vi "Generator.vi"() -> ()   [LabVIEW 2018]
uses:
  <instrlib>/Siglent SDG X Series/Siglent SDG X Series.lvlib
panel:
  in  "Filename":string="1"
  in  "File Directory":path
  out "Output Directory":path
  in  "format string":string="Channel: %g \nWavetype: %g \nAMP: %gV\nFreq: %gHz \nRiseTime: %gs \nFallTime: %gs \nDutyCycle: %g"
  out "error out 2":errorcluster
  out "Output Filename":path
  out "error out":errorcluster
  out "VISA resource name out":refnum<visa-resource-name>
  in  "True To \ngenerate\n pulse":bool
  in  "Rise (20 ns)":dbl=1.04e-08 format="%#.3g"
  in  "Delay (0.00 s)":dbl min=-1000000.0 max=1000000.0
  in  "Duty (20%)":dbl=4.32 min=0.0001 max=100.0 format="%.4g"
  in  "Fall (20 ns)":dbl=8.4e-09 format="%#.3g"
  in  "Phase (0.0 degrees)":dbl=0.002 min=-360.0 max=360.0 format="%#.1g"
  in  "Waveform Function (0: Sine) in":u16(ring) items=["Sine", "Square", "Ramp", "DC", "Pulse", "Arb"]
  in  "DC Offset (0.00 V) in":dbl
  in  "Frequency (1000 Hz)":dbl=1500000.0 format="%#.6g"
  in  "Amplitude (1.0 Vpp)":dbl=1.0 format="%#.3f"
  in  "Enable Output (T: Enable)":bool=TRUE
  in  "Channel (1:Channel 1)":i32(ring)=1 items=["Channel 1"=1, "Channel 2"=2]
  in  "VISA Refnum in":refnum<visa-resource-name>="USB0::0xF4EC::0xEE38::SDG2XCAD2R3765::INSTR"
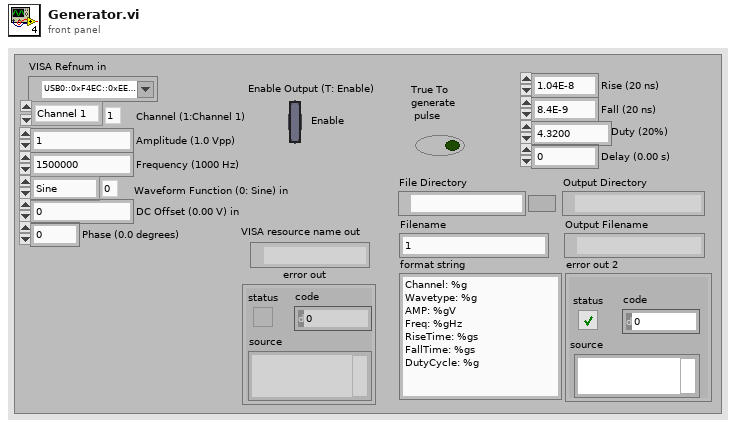
[diagram p1: front panel]
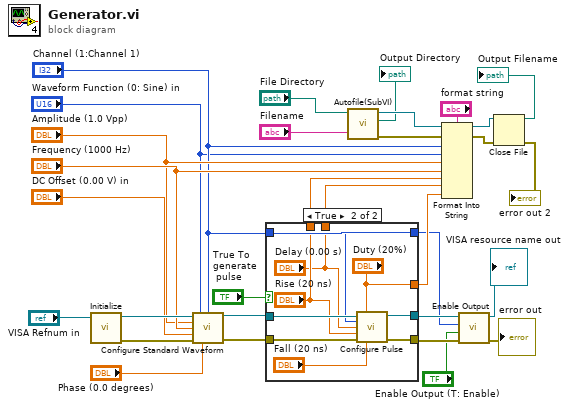
[diagram p0: block diagram]
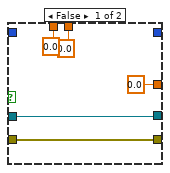
[diagram p2: hidden frame]
diagram:
  n1 = call <instrlib>:"Initialize.vi"("VISA resource name"="VISA Refnum in") -> ("error out"=w25:errorcluster, "VISA resource name out"=w26:refnum<visa-resource-name>)  [unwired: 9 in]
  n2 = call <instrlib>:"Configure Standard Waveform.vi"("VISA resource name"=w26, "Waveform Function (0: Sine)"="Waveform Function (0: Sine) in", "Channel (1:Channel 1)"="Channel (1:Channel 1)", "Amplitude (1.0 Vpp)"="Amplitude (1.0 Vpp)", "Frequency (1000 Hz)"="Frequency (1000 Hz)", "DC Offset (0.00 V)"="DC Offset (0.00 V) in", "error in (no error)"=w25, "Phase (0.0 degrees)"="Phase (0.0 degrees)") -> ("VISA resource name out"=w21:refnum<visa-resource-name>, "error out"=w24:errorcluster)  [unwired: 6 in]
  n3 = case shown="True" "True To \ngenerate\n pulse" {
    tunnel: [w35 w43] -> w30
    tunnel: [w34 w42] -> w29
    tunnel: w21 -> [w35 w41]
    tunnel: w24 -> [w34 w40]
    tunnel: "Channel (1:Channel 1)" -> [_ w39]
    tunnel: "Channel (1:Channel 1)" -> [_ _]
    tunnel: [0.0 ("Duty (20%)") "Duty (20%)"] -> w17
    tunnel: [0.0 ("Rise (20 ns)") "Rise (20 ns)"] -> w9
    tunnel: [0.0 ("Delay (0.00 s)") "Delay (0.00 s)"] -> w8
    frame False {
    }
    frame True {
      n4 = call <instrlib>:"Configure Pulse.vi"("VISA resource name"=w41, "Duty (20%)"="Duty (20%)", "Channel (1:Channel 1)"=w39, "Delay (0.00 s)"="Delay (0.00 s)", "Rise (20 ns)"="Rise (20 ns)", "error in (no error)"=w40, "Fall (20 ns)"="Fall (20 ns)") -> ("VISA resource name out"=w43:refnum<visa-resource-name>, "error out"=w42:errorcluster)  [unwired: 7 in]
    }
  }
  n5 = call "Autofile(SubVI).vi"("Filename"="Filename", "File Directory"="File Directory") -> ("error out"=w4:errorcluster, "Output Directory"=→"Output Directory":path, "Byte Stream File out"=w5:refnum<file>)  [unwired: 7 in]
  n6 = Format Into String(format string="format string", initial string=w5, error in=w4, "Channel (1:Channel 1)", "Waveform Function (0: Sine) in", "Amplitude (1.0 Vpp)", "Frequency (1000 Hz)", w9, w8, w17) -> (resulting string=w16:refnum<file>, error out=w13:errorcluster)
  n7 = call <instrlib>:"Enable Output.vi"("error in (no error)"=w29, "Enable Output (T: Enable)"="Enable Output (T: Enable)", "Channel (1:Channel 1)"="Channel (1:Channel 1)", "VISA resource name"=w30) -> ("error out"=→"error out":errorcluster, "VISA resource name out"=→"VISA resource name out":refnum<visa-resource-name>)  [unwired: 6 in]
  n8 = Close File(refnum=w16, error in=w13) -> (path=→"Output Filename":path, error out=→"error out 2":errorcluster)
